vi "SerialUltra.vi"(8 "error in":errorcluster, 9 "State":T1=enum."Init", 10 "Data Write":string, 11 "IN COM":refnum<visa-resource-name>) -> (0 "error out":errorcluster, 1 "IsData":bool, 2 "DataOut":string, 3 "OUT COM 2":refnum<visa-resource-name>, 4 "Is Connected":bool)   [LabVIEW 2017]
uses:
  stateSerialUltra.ctl
  <vilib>/Instr/_visa.llb/VISA Configure Serial Port (Instr).vi
panel:
  in  "termination char\n(0xA = '\\n' = LF)":u8=10 format="%.0x"
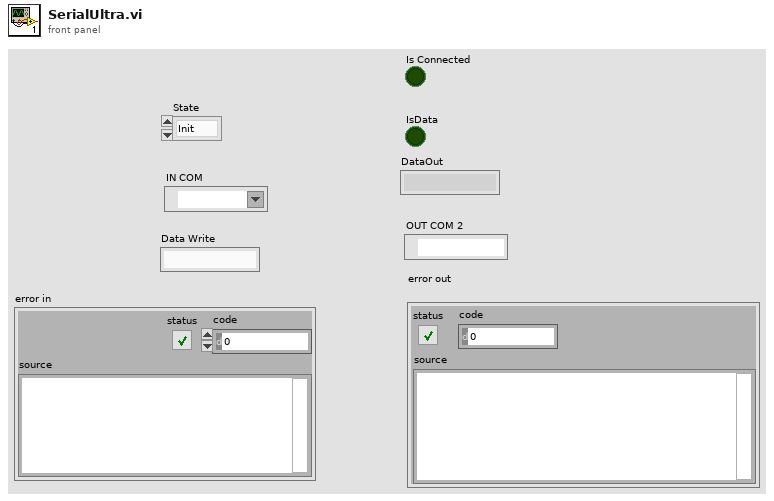
[diagram p1: front panel]
types:
  T1 = typedef "stateSerialUltra.ctl" = enum16{"findCOM", "Init", "CheckConnect", "Read", "Write", "exit"}
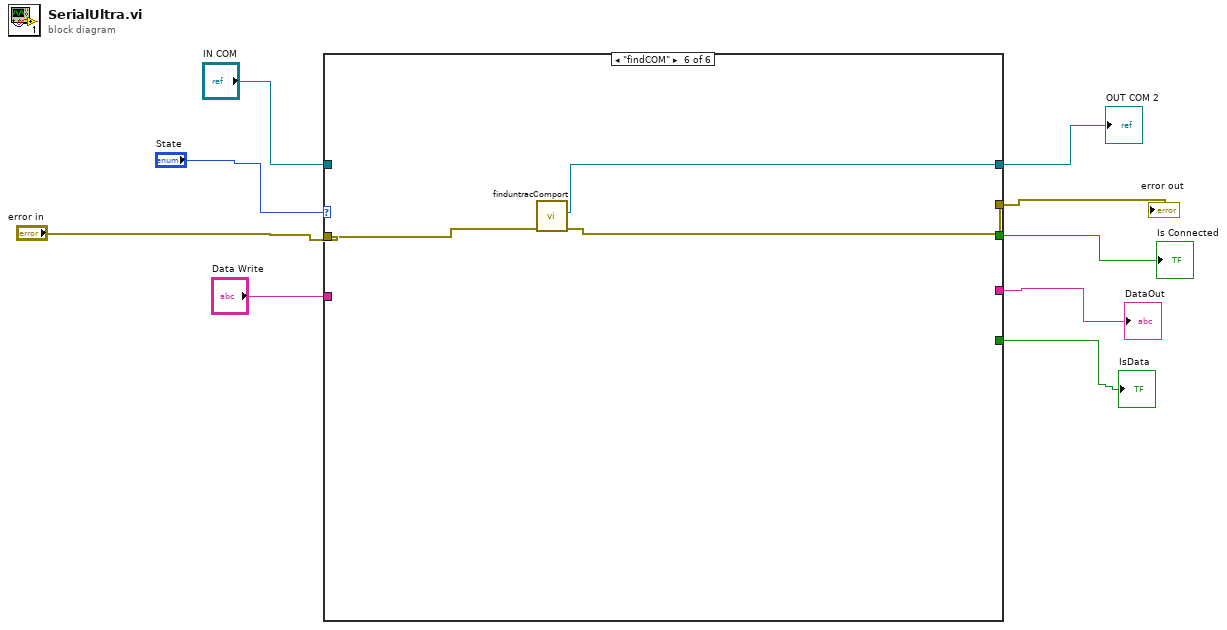
[diagram p0: block diagram]
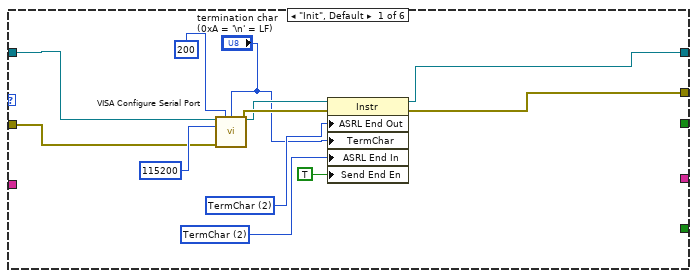
[diagram p2: hidden frame]
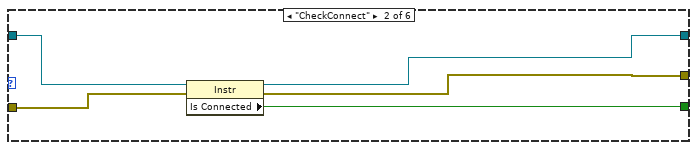
[diagram p3: hidden frame]
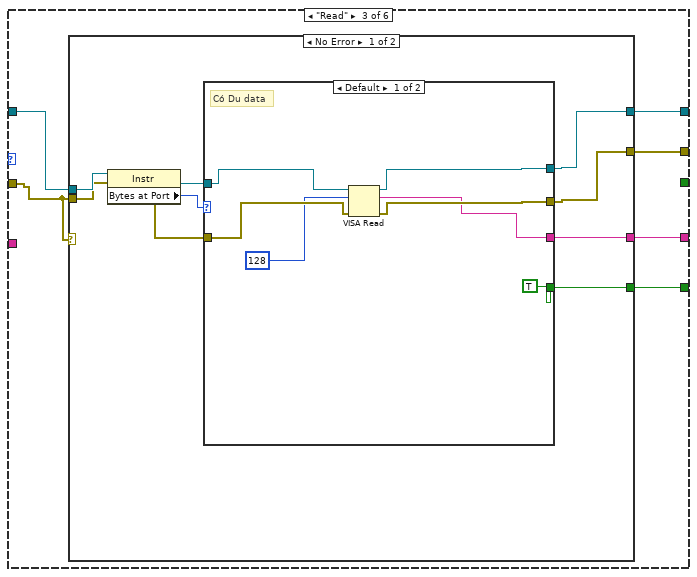
[diagram p4: hidden frame]
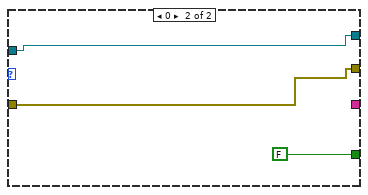
[diagram p5: hidden frame]
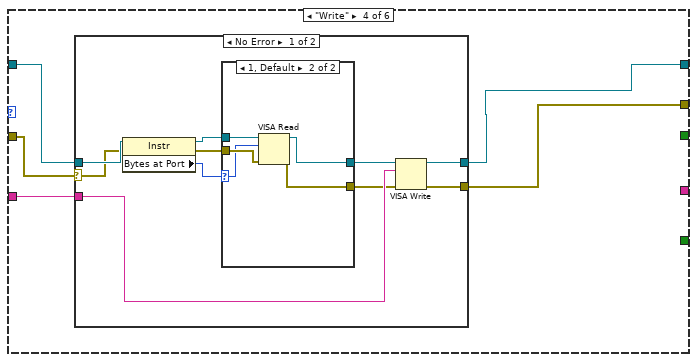
[diagram p7: hidden frame]
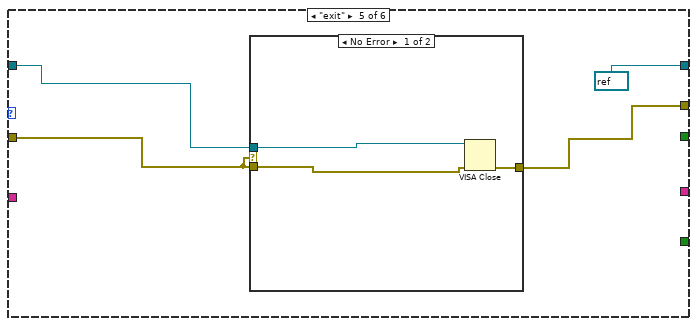
[diagram p10: hidden frame]
diagram:
  n1 = case shown="\"findCOM\"" "State" {
    tunnel: [w11 w23 w30 w57 refnum<visa-resource-name> refnum ("OUT COM") w88] -> w1
    tunnel: [w10 w24 w31 w56 w81 w87] -> w7
    tunnel: "error in" -> [w17 w25 w27 w55 w78 w86]
    tunnel: "IN COM" -> [w18 w26 w32 w54 w80 _]
    tunnel: [_ w22 _ _ _ _] -> w6
    tunnel: "Data Write" -> [_ _ _ w58 _ _]
    tunnel: [_ _ w29 _ _ _] -> w4
    tunnel: [_ _ w28 _ _ _] -> w3
    frame "Init", Default {
      w13 = u16 2 items=["None", "Last Bit", "TermChar"] ("Serial Settings:End Mode for Reads")
      w20 = u16 2 items=["None", "Last Bit", "TermChar", "Break"] ("Serial Settings:End Mode for Writes")
      n2 = call-poly "VISA Configure Serial Port"("VISA resource name"=w18, "timeout (10sec)"=u32 200, "termination char\n(0xA = '\\n' = LF)"="termination char\n(0xA = '\\n' = LF)", "baud rate (9600)"=u32 115200, "error in (no error)"=w17) -> ("VISA resource name out"=w15:refnum<visa-resource-name>, "error out"=w16:errorcluster)  [unwired: 9 in]
      n3 = property class="Instr"(reference=w15, error in=w16, "ASRL End Out"=w20, "TermChar"="termination char\n(0xA = '\\n' = LF)", "ASRL End In"=w13, "Send End En"=TRUE ("Message Based Settings:Send End Enable")) -> (reference out=w11:refnum<visa-resource-name>, error out=w10:errorcluster)
    }
    frame "CheckConnect" {
      n4 = property class="Instr"(reference=w26, error in=w25) -> (reference out=w23:refnum<visa-resource-name>, error out=w24:errorcluster, "Is Connected"=w22:bool)
    }
    frame "Read" {
      n5 = case shown="No Error" w27 {
        tunnel: w32 -> [w39 w53]
        tunnel: w27 -> [w38 w52]
        tunnel: [w37 w52] -> w31
        tunnel: [w36 w53] -> w30
        tunnel: [w35 _] -> w29
        tunnel: [w33 _] -> w28
        frame No Error {
          n6 = property class="Instr"(reference=w39, error in=w38) -> (reference out=w41:refnum<visa-resource-name>, error out=w40:errorcluster, "Bytes at Port"=w34:u32)
          n7 = case shown="Default" w34 {
            tunnel: w41 -> [w46 w51]
            tunnel: w40 -> [w45 w50]
            tunnel: [w47 w50] -> w37
            tunnel: [w48 w51] -> w36
            tunnel: [w42 _] -> w35
            tunnel: [TRUE ("Is Connected 2") FALSE ("Is Connected 2")] -> w33
            frame Default {
              # "Có Du data"
              n8 = VISA Read(VISA resource name=w46, byte count=u32 128, error in (no error)=w45) -> (VISA resource name out=w48:refnum<visa-resource-name>, read buffer=w42:string, error out=w47:errorcluster)  [unwired: 1 out]
            }
            frame 0 {
            }
          }
        }
        frame Error {
        }
      }
    }
    frame "Write" {
      n9 = case shown="No Error" w55 {
        selector: w55 -> [w65 w76]
        tunnel: w54 -> [w66 w77]
        tunnel: w58 -> [w64 _]
        tunnel: [w68 w77] -> w57
        tunnel: [w67 w76] -> w56
        frame No Error {
          n10 = property class="Instr"(reference=w66, error in=w65) -> (reference out=w63:refnum<visa-resource-name>, error out=w62:errorcluster, "Bytes at Port"=w61:u32)
          n11 = case shown="1, Default" w61 {
            selector: w61 -> [_ w71]
            tunnel: w63 -> [w70 w75]
            tunnel: w62 -> [w69 w74]
            tunnel: [w70 w73] -> w60
            tunnel: [w69 w72] -> w59
            frame 0 {
            }
            frame 1, Default {
              n12 = VISA Read(VISA resource name=w75, byte count=w71, error in (no error)=w74) -> (VISA resource name out=w73:refnum<visa-resource-name>, error out=w72:errorcluster)  [unwired: 2 out]
            }
          }
          n13 = VISA Write(VISA resource name=w60, write buffer=w64, error in (no error)=w59) -> (VISA resource name out=w68:refnum<visa-resource-name>, error out=w67:errorcluster)  [unwired: 1 out]
        }
        frame Error {
        }
      }
    }
    frame "exit" {
      n14 = case shown="No Error" w78 {
        tunnel: w78 -> [w82 w85]
        tunnel: [w84 w85] -> w81
        tunnel: w80 -> [w83 _]
        frame No Error {
          n15 = VISA Close(VISA resource name=w83, error in (no error)=w82) -> (error out=w84:errorcluster)
        }
        frame Error {
        }
      }
    }
    frame "findCOM" {
      n16 = call "finduntracComport.vi"("error IN"=w86) -> ("OUT COM"=w88:refnum<visa-resource-name>, "error out"=w87:errorcluster)  [unwired: 8 in]
    }
  }
  "error out" <- w7
  "Is Connected" <- w6
  "DataOut" <- w4
  "IsData" <- w3
  "OUT COM 2" <- w1
